vi "Listbox Text Wrapper.vi"(10 "Size:Width":u32, 11 "Input Text":string) -> (3 "Wrapped Text":string)   [LabVIEW 2014]
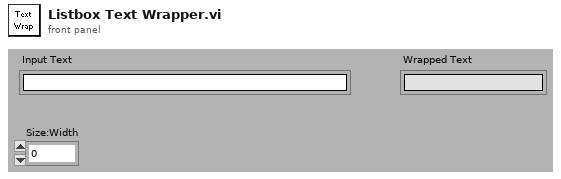
[diagram p1: front panel]
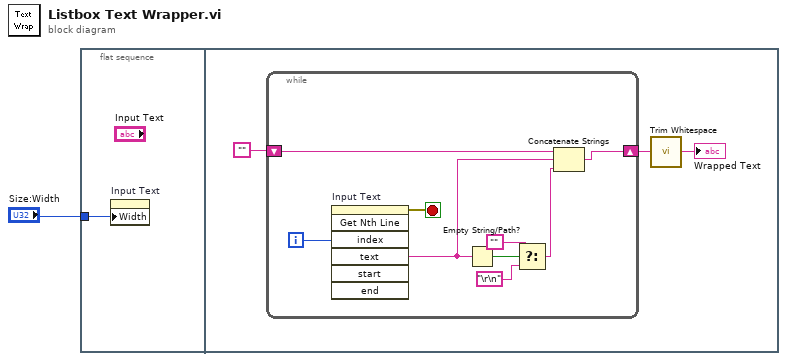
[diagram p0: block diagram]
diagram:
  n1 = flat-sequence {
    tunnel: "Size:Width" -> [w2]
    frame #0 {
      n2 = property on="Input Text" class="Str"("Width"=w2) -> ()  [unwired: 2 in, 2 out]
    }
    frame #1 {
      n3 = while {
        shift-right: [w7] -> w4
        shift-left: "" -> [w10]
        i -> [w6]
        stop <- w14 stop-if-true
        n4 = invoke on="Input Text" class="Str" method="Get Nth Line"("index"=w6) -> (error out=w14:errorcluster, "text"=w9:string)  [unwired: 6 in, 5 out]
        n5 = Empty String/Path?(string/path=w9) -> (empty?=w12:bool)
        n6 = Select(t="", s=w12, f="\r\n") -> (s? t:f=w8:string)
        n7 = Concatenate Strings(w10, w9, w8) -> (w7:string)
      }
      n8 = call <vilib>:"Trim Whitespace.vi"("string"=w4) -> ("trimmed string"=→"Wrapped Text":string)  [unwired: 1 in]
    }
  }
